vi "Exemplo 2.vi"() -> ()   [LabVIEW 2021]
uses:
  <vilib>/Analysis/3filter.llb/Butterworth Filter (DBL).vi
  <vilib>/Utility/file.llb/Write Delimited Spreadsheet (DBL).vi
  <vilib>/measure/NI_MABase.lvlib
  <vilib>/Analysis/NI_AALBase.lvlib
  <vilib>/ptbypt/NI_PtbyPt.lvlib
panel:
  out "x/y":dbl
  out "XY Graph":T1(graph)
  in  "y":dbl
  out "Tempo de Execução":i64
  out "Gauge":dbl(knob) scale=0.0..1000.0
  out "max value":dbl
  in  "low cutoff freq: fl":dbl=0.12500000000000006 format="%0.4f"
  in  "high cutoff freq: fh":dbl=0.45000000000000007 format="%0.2f"
  out "Waveform Graph 4":dbl[](graph)
  out "Waveform Graph 3":dbl[](graph)
  out "t0":timestamp
  out "Waveform Graph 2":dbl[](graph)
  out "Waveform Graph":dbl[](graph)
  in  "stop":bool
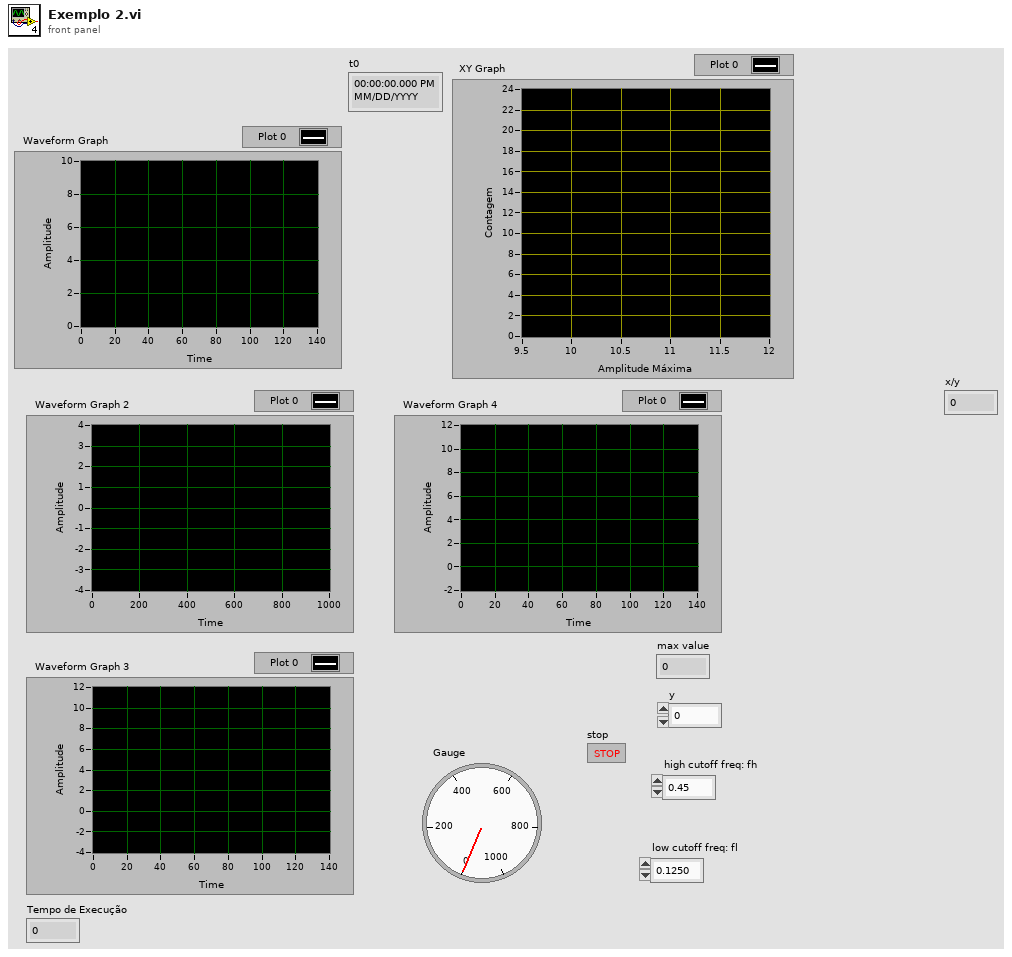
[diagram p1: front panel]
types:
  T1 = cluster{"X Values":dbl[], "Histogram: h(x)":i32[]}
  T2 = enum16{"open", "replace", "create", "open or create", "replace or create", "replace or create with confirmation"}
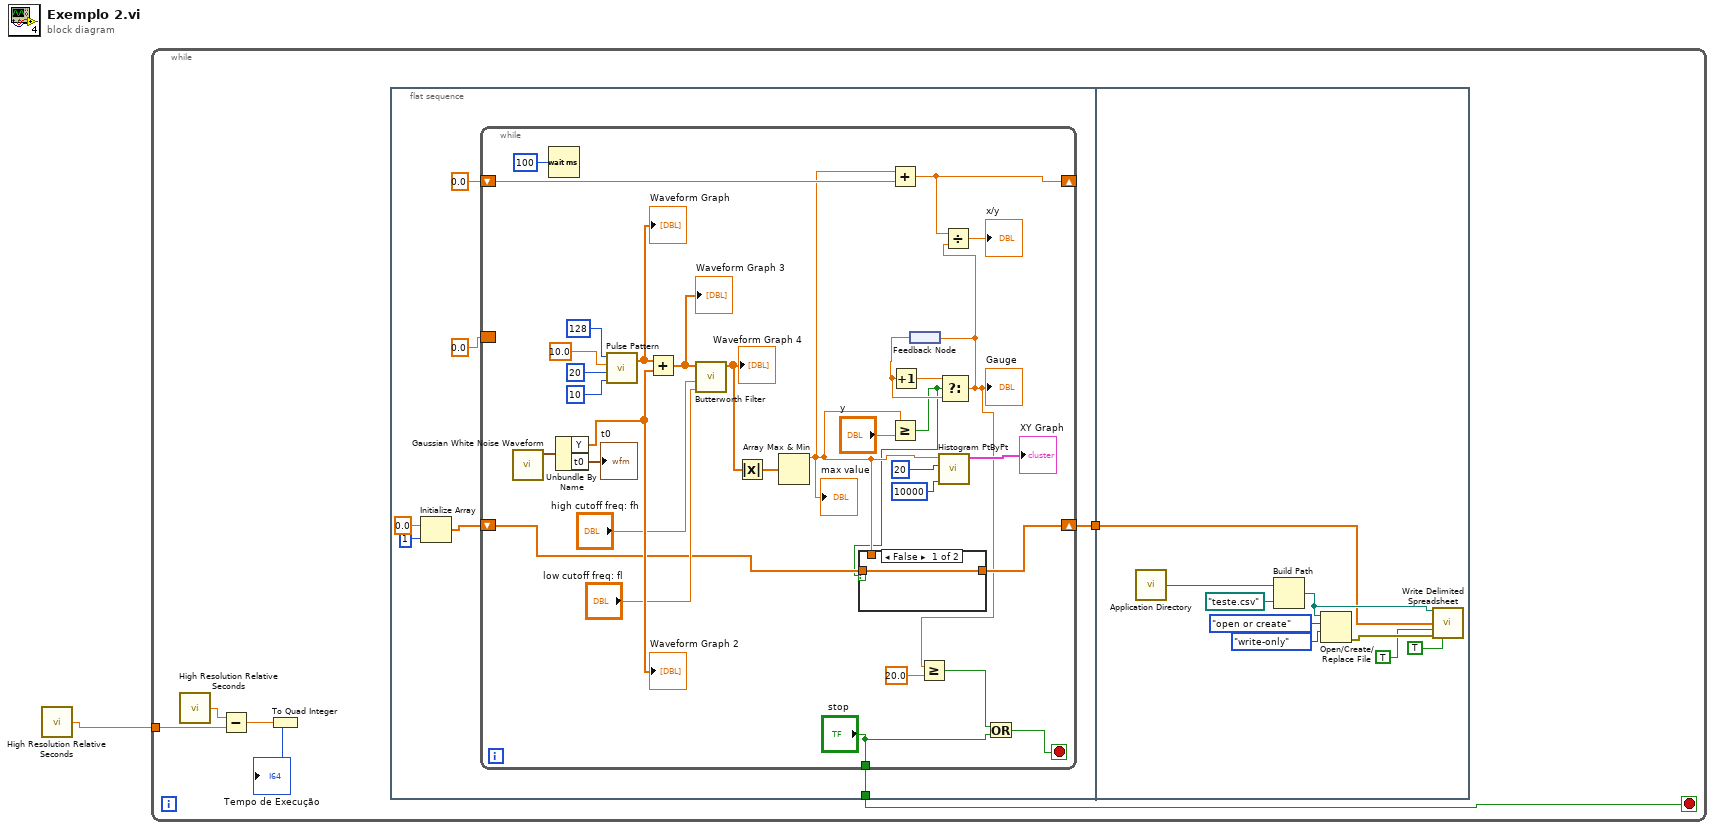
[diagram p0: block diagram]
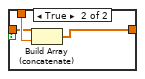
[diagram p2: hidden frame]
diagram:
  n1 = call <vilib>:"High Resolution Relative Seconds.vi"() -> ("relative seconds"=w1:dbl)
  n2 = while {
    tunnel: w1 -> [w4]
    stop <- w2 stop-if-true
    n3 = call <vilib>:"High Resolution Relative Seconds.vi"() -> ("relative seconds"=w7:dbl)
    n4 = Subtract(x=w7, y=w4) -> (x-y=w6:dbl)
    n5 = To Quad Integer(1:w6) -> (0:→"Tempo de Execução":i64)
    n6 = flat-sequence {
      tunnel: [w12] -> w3
      tunnel: [w11] -> w2
      tunnel: w3 -> [w52]
      frame #0 {
        n7 = Initialize Array(0.0 ("element"), 1 ("dimension size")) -> (w10:dbl[])
        n8 = while {
          shift-right: [w26] -> _
          shift-left: 0.0 -> [w27]
          shift-right: [w22] -> w12
          shift-left: w10 -> [w21]
          border: 0.0 -> [_]
          tunnel: ["stop"] -> w11
          stop <- w19 stop-if-true
          n9 = call <vilib>:"Gaussian White Noise Waveform.vi"() -> ("signal out"=w45:waveform(dbl))  [unwired: 10 in, 1 out]
          n10 = Wait (ms)(milliseconds to wait=u32 100) -> ()  [unwired: 1 out]
          n11 = Unbundle By Name(w45) -> ("Y"=w43:dbl[], "t0"=→"t0":timestamp)
          "Waveform Graph 2" <- w43
          n12 = call <vilib>:"Pulse Pattern.vi"("width"=10, "delay"=20, "amplitude"=10.0, "samples"=128) -> ("Pulse Pattern"=w35:dbl[])  [unwired: 1 out]
          "Waveform Graph" <- w35
          n13 = Add(x=w35, y=w43) -> (x+y=w42:dbl[])
          "Waveform Graph 3" <- w42
          n14 = call-poly <vilib>:"Butterworth Filter.vi"("low cutoff freq: fl"="low cutoff freq: fl", "high cutoff freq: fh"="high cutoff freq: fh", "X"=w42) -> ("Filtered X"=w39:dbl[])  [unwired: 5 in, 1 out]
          "Waveform Graph 4" <- w39
          n15 = Absolute Value(x=w39) -> (abs(x)=w37:dbl[])
          n16 = Array Max & Min(array=w37) -> (max value=w23:dbl)  [unwired: 3 out]
          "max value" <- w23
          n17 = Add(x=w23, y=w27) -> (x+y=w26:dbl)
          n18 = Greater Or Equal?(x=w23, y="y") -> (x >= y?=w20:bool)
          n19 = case shown="False" w20 {
            tunnel: w23 -> [_ w50]
            tunnel: [w47 w49] -> w22
            tunnel: w21 -> [w47 w48]
            frame False {
            }
            frame True {
              n20 = Build Array (concatenate)(w48, w50) -> (w49:dbl[])
            }
          }
          n21 = feedback #1() -> (w25:dbl)
          n22 = Increment(x=w25) -> (x+1=w38:dbl)
          n23 = call <vilib>:"Histogram PtByPt.vi"("sample length"=10000, "intervals"=20, "x"=w23) -> ("Histogram Graph"=→"XY Graph":T1)  [unwired: 5 in, 3 out]
          n24 = Select(t=w38, s=w20, f=w25) -> (s? t:f=w16:dbl)
          "Gauge" <- w16
          n25 = feedback-in #1(w16) -> ()
          n26 = Greater Or Equal?(x=w16, y=20.0) -> (x >= y?=w17:bool)
          n27 = Divide(x=w26, y=w16) -> (x/y=→"x/y":dbl)
          n28 = Or(x=w17, y="stop") -> (x .or. y?=w19:bool)
        }
      }
      frame #1 {
        n29 = call <vilib>:"Application Directory.vi"() -> ("Application Directory"=w59:path)
        n30 = Build Path(base path=w59, name or relative path=path "teste.csv") -> (appended path=w57:path)
        n31 = Open/Create/Replace File(file path (use dialog)=w57, operation (0:open)=T2."open or create", access (0:read/write)=enum16{"read/write", "read-only", "write-only"}."write-only") -> (error out=w58:errorcluster)  [unwired: 3 in, 2 out]
        n32 = call-poly <vilib>:"Write Delimited Spreadsheet.vi"("file path (dialog if empty)"=w57, "1D data"=w52, "append to file? (new file:F)"=TRUE, "error in (no error)"=w58, "transpose? (no:F)"=TRUE) -> ()  [unwired: 9 in, 2 out]
      }
    }
  }
